vi "Salva_systems_messages.vi"(5 "Mensagem":string) -> ()   [LabVIEW 2018, in "Shared_160.lvlib"]
uses:
  Shared_160.lvlib
panel:
  out "date string":string
  out "String":string
  out "Comando":string
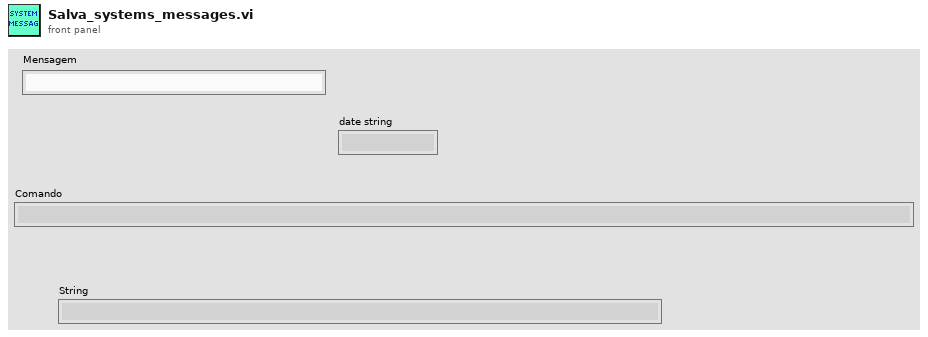
[diagram p1: front panel]
types:
  T1 = enum16{"open", "open or create", "create or replace", "create"}
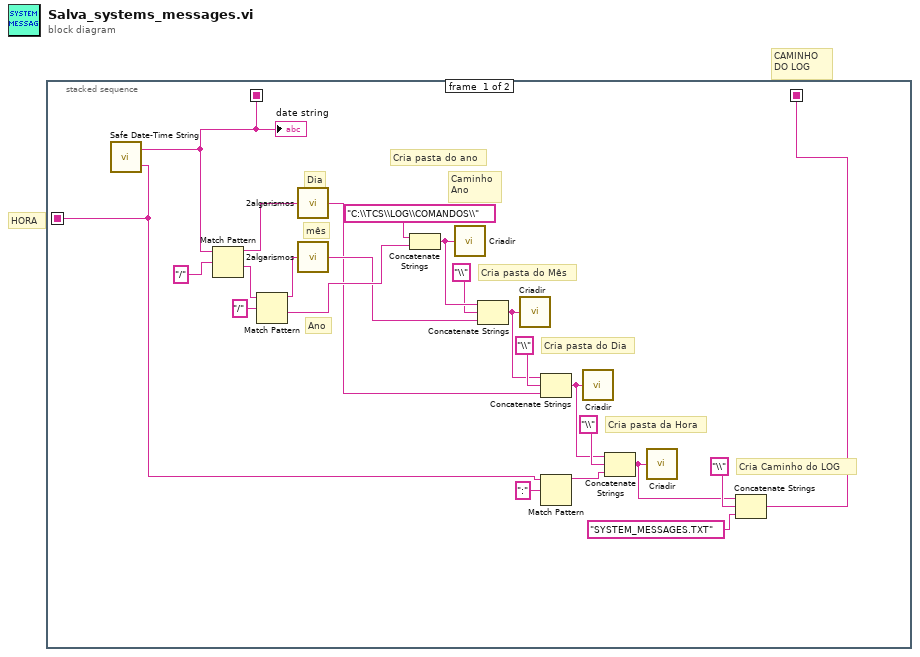
[diagram p0: block diagram]
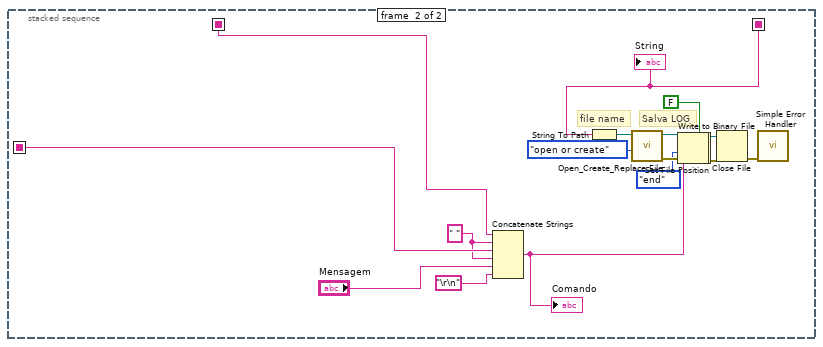
[diagram p2: hidden frame]
diagram:
  # "HORA"
  # "CAMINHO\nDO LOG"
  n1 = stacked-sequence {
    seq-local: [w8 _] -> [_ w40]
    seq-local: [w2 _] -> [_ w38]
    seq-local: [w1 _] -> [_ w36]
    frame #0 {
      # "Cria pasta da Hora"
      # "Cria Caminho do LOG"
      # "Cria pasta do Dia"
      # "Cria pasta do Mês"
      # "Caminho\nAno"
      # "Ano"
      # "mês"
      # "Dia"
      # "Cria pasta do ano"
      n2 = call "Safe Date-Time String.vi"() -> ("Safe time string"=w2:string, "Safe date string"=w1:string)  [unwired: 2 in, 1 out]
      "date string" <- w1
      n3 = Match Pattern(string=w1, regular expression="/") -> (before substring=w20:string, after substring=w21:string)  [unwired: 1 in, 2 out]
      n4 = Match Pattern(string=w21, regular expression="/") -> (before substring=w19:string, after substring=w17:string)  [unwired: 1 in, 2 out]
      n5 = call "2algarismos.vi"("entrada"=w20) -> ("saida"=w11:string)
      n6 = call "2algarismos.vi"("entrada"=w19) -> ("saida"=w14:string)
      n7 = Concatenate Strings("C:\\TCS\\LOG\\COMANDOS\\" ("SOMENTE DIRETORIO"), w17) -> (w16:string)
      n8 = call "Criadir.vi"("SOMENTE DIRETORIO"=w16) -> ()  [unwired: 2 out]
      n9 = Concatenate Strings(w16, "\\" ("regular expression"), w14) -> (w12:string)
      n10 = call "Criadir.vi"("SOMENTE DIRETORIO"=w12) -> ()  [unwired: 2 out]
      n11 = Concatenate Strings(w12, "\\" ("regular expression"), w11) -> (w6:string)
      n12 = Match Pattern(string=w2, regular expression=":") -> (before substring=w4:string)  [unwired: 1 in, 3 out]
      n13 = call "Criadir.vi"("SOMENTE DIRETORIO"=w6) -> ()  [unwired: 2 out]
      n14 = Concatenate Strings(w6, "\\" ("regular expression"), w4) -> (w3:string)
      n15 = call "Criadir.vi"("SOMENTE DIRETORIO"=w3) -> ()  [unwired: 2 out]
      n16 = Concatenate Strings(w3, "\\" ("regular expression"), "SYSTEM_MESSAGES.TXT" ("regular expression")) -> (w8:string)
    }
    frame #1 {
      w24 = " " ("date string")
      # "Salva LOG"
      # "file name"
      n17 = Concatenate Strings(w36, w24, w38, w24, "Mensagem", "\r\n") -> (w41:string)
      "Comando" <- w41
      n18 = String To Path(string=w40) -> (path=w28:path)
      n19 = call <vilib>:"Open_Create_Replace File.vi"("function (open:0)"=T1."open or create", "file path"=w28) -> ("error out"=w31:errorcluster, "refnum"=w34:refnum<file>)  [unwired: 6 in, 2 out]
      n20 = Set File Position(refnum=w34, from (0:start)=enum16{"start", "end", "current"}."end" ("pos mode (0:2)"), error in=w31) -> (refnum out=w27:refnum<file>, error out=w26:errorcluster)  [unwired: 1 in]
      n21 = Write to Binary File(file (use dialog)=w27, data=w41, error in=w26, 5:FALSE ("prepend array or string size? (T)")) -> (refnum out=w33:refnum<file>, error out=w32:errorcluster)  [unwired: 2 in, 1 out]
      n22 = Close File(refnum=w33, error in=w32) -> (error out=w35:errorcluster)  [unwired: 1 out]
      n23 = call <vilib>:"Simple Error Handler.vi"("error in (no error)"=w35) -> ()  [unwired: 4 in, 5 out]
      "String" <- w40
    }
  }
